vi "ColorTableGenerator.vi"() -> (0 "?":u32[](array[colorbox]))   [LabVIEW 2025]
doc: "Color Table Generator.vi is a subVI called by Color Table Example.vi\n\nThis VI generates a color table based on the beginning, middle, and end RGB color combinations the user specifies. Using an XY graph and cursors, the user mixes red, green, and blue components to create the start, middle, and end color combinations for the color table.\nAuthor: Scott Hannahs <sth@magnet.fsu.edu>\n\nThis software is licensed for use under the “MIT License\"\nCopyright (c) 2025 Scott Hannahs, sth@sth@magnet.sthnet.net\n\nPermission is hereby granted, free of charge, to any person obtaining a copy of this software and associated documentation files (the \"Software\"), to deal in the Software without restriction, including without limitation the rights to use, copy, modify, merge, publish, distribute, sublicense, and/or sell copies of the Software, and to permit persons to whom the Software is furnished to do so, subject to the following conditions: The above copyright notice and this permission notice shall be included in all copies or substantial portions of the Software.\n\nTHE SOFTWARE IS PROVIDED \"AS IS\", WITHOUT WARRANTY OF ANY KIND, EXPRESS OR IMPLIED, INCLUDING BUT NOT LIMITED TO THE WARRANTIES OF MERCHANTABILITY, FITNESS FOR A PARTICULAR PURPOSE AND NONINFRINGEMENT. IN NO EVENT SHALL THE AUTHORS OR COPYRIGHT HOLDERS BE LIABLE FOR ANY CLAIM, DAMAGES OR OTHER LIABILITY, WHETHER IN AN ACTION OF CONTRACT, TORT OR OTHERWISE, ARISING FROM, OUT OF OR IN CONNECTION WITH THE SOFTWARE OR THE USE OR OTHER DEALINGS IN THE SOFTWARE."
panel:
  in  "Out of range below\n(color 0)":u32(colorbox)
  in  "Out of range above\n(color 255)":u32(colorbox)=16711680
  in  "Cancel":bool
  in  "Accept":bool
  in  "final color":cluster{u8, u8, u8}(slide)={255, 234, 0} scale=0.0..255.0
  in  "beginning color":cluster{u8, u8, u8}(slide)={0, 21, 255} scale=0.0..255.0
  out "?":cluster{u8[]}[](graph)
  # "Use the two sliders\nand the cursors to\ndefine the color table."
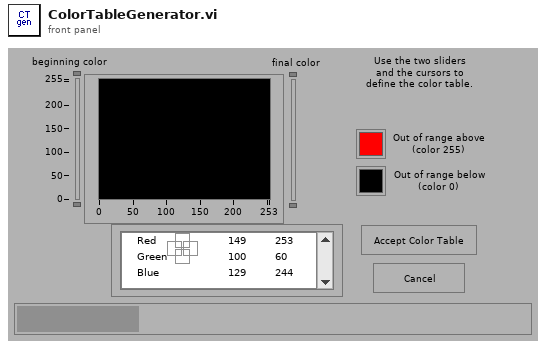
[diagram p1: front panel]
types:
  T1 = cluster{u8, u8, "Cursor.Cursor Y":dbl, "Cursor.Cursor X":dbl}
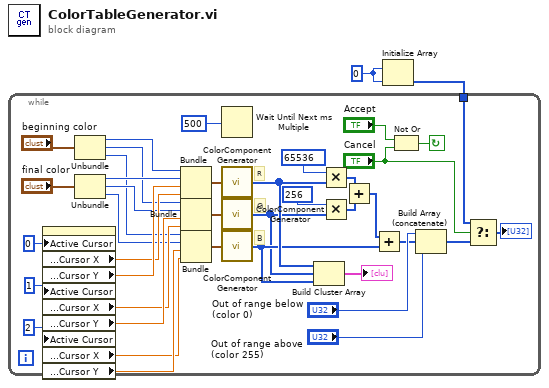
[diagram p0: block diagram]
diagram:
  w2 = u32 0
  n1 = Initialize Array(w2, w2) -> (w1:u32[])
  n2 = while {
    tunnel: w1 -> [w14]
    stop <- w15 continue-if-true
    # "B"
    # "G"
    # "R"
    n3 = property class="WFGraph (strict)"("Active Cursor"=0, "Active Cursor"=1, "Active Cursor"=2) -> ("Cursor.Cursor Position:Cursor X"=w36:dbl, "Cursor.Cursor Position:Cursor Y"=w37:dbl, "Cursor.Cursor Position:Cursor X"=w38:dbl, "Cursor.Cursor Position:Cursor Y"=w39:dbl, "Cursor.Cursor Position:Cursor X"=w40:dbl, "Cursor.Cursor Position:Cursor Y"=w41:dbl)  [unwired: 2 in, 2 out]
    n4 = Unbundle("beginning color") -> (w30:u8, w31:u8, w32:u8)
    n5 = Unbundle("final color") -> (w33:u8, w34:u8, w35:u8)
    n6 = Bundle(w30, w33, "Cursor.Cursor Y"=w37, "Cursor.Cursor X"=w36) -> (w27:T1)  [unwired: 1 in]
    n7 = Bundle(w31, w34, "Cursor.Cursor Y"=w39, "Cursor.Cursor X"=w38) -> (w10:T1)  [unwired: 1 in]
    n8 = Bundle(w32, w35, "Cursor.Cursor Y"=w41, "Cursor.Cursor X"=w40) -> (w9:T1)  [unwired: 1 in]
    n9 = Wait Until Next ms Multiple(millisecond multiple=500) -> ()  [unwired: 1 out]
    n10 = call "ColorComponentGenerator.vi"("Component definition"=w27) -> ("Component array"=w23:u8[])
    n11 = call "ColorComponentGenerator.vi"("Component definition"=w10) -> ("Component array"=w7:u8[])
    n12 = call "ColorComponentGenerator.vi"("Component definition"=w9) -> ("Component array"=w8:u8[])
    n13 = Build Cluster Array(w23, w7, w8) -> (→"?":cluster{"Component array":u8[]}[])
    n14 = Multiply(x=u32 65536, y=w23) -> (x*y=w20:u32[])
    n15 = Multiply(x=u32 256, y=w7) -> (x*y=w19:u32[])
    n16 = Add(x=w20, y=w19) -> (x+y=w21:u32[])
    n17 = Add(x=w21, y=w8) -> (x+y=w3:u32[])
    n18 = Not Or(1:"Cancel", 2:"Accept") -> (0:w15:bool)
    n19 = Build Array (concatenate)("Out of range below\n(color 0)", w3, "Out of range above\n(color 255)") -> (w6:u32[])
    n20 = Select(t=w14, s="Cancel", f=w6) -> (s? t:f=→"?":u32[])
  }
